vi "sub-GetLanguageInfo.vi"() -> (2 "selected":i32, 3 "languages":cluster{string, "appended path":path, string}[](array[cluster]))   [LabVIEW 2011]
uses:
  <vilib>/Utility/config.llb/Read Key (I32).vi
  <vilib>/Utility/config.llb/Read Key (String).vi
  <vilib>/Utility/config.llb/NI_LVConfig.lvlib
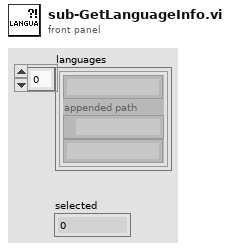
[diagram p1: front panel]
types:
  T1 = typedef "NI_LVConfig.lvlib/Config Data RefNum.ctl" = refnum<k1>
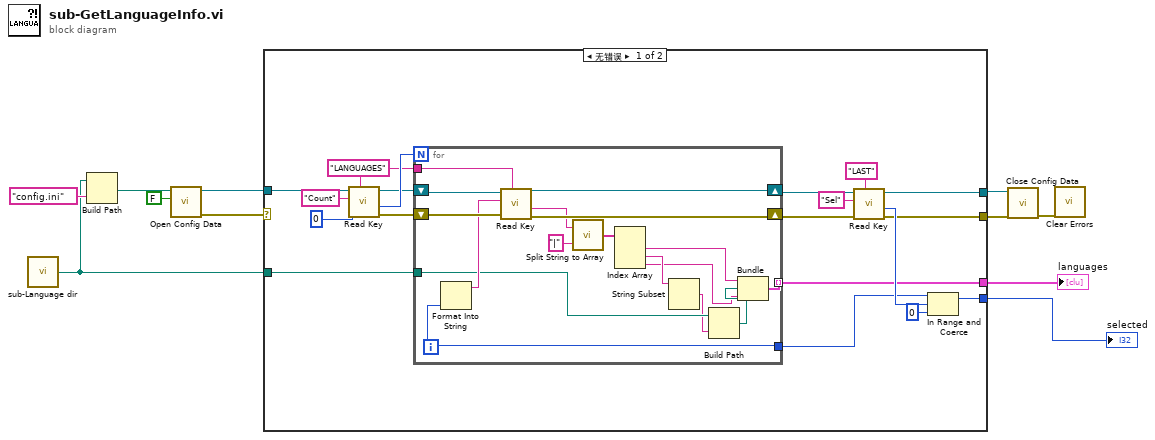
[diagram p0: block diagram]
diagram:
  n1 = call "sub-Language dir.vi"() -> ("folder"=w2:path)
  n2 = Build Path(base path=w2, name or relative path="config.ini" ("名称或相对路径")) -> (appended path=w10:path)
  n3 = call <vilib>:"Open Config Data.vi"("create file if necessary (T)"=FALSE, "configuration file path"=w10) -> ("error out"=w8:errorcluster, "refnum"=w7:T1)  [unwired: 7 in, 1 out]
  n4 = case shown="无错误" w8 {
    selector: w8 -> [_ w48]
    tunnel: w7 -> [w30 w49]
    tunnel: [w16 _] -> w3
    tunnel: [w15 _] -> w1
    tunnel: [w14 w49] -> w5
    tunnel: [w13 w48] -> w6
    tunnel: w2 -> [w12 _]
    frame No Error {
      w24 = "LANGUAGES" ("section")
      n5 = call-poly <vilib>:"Read Key.vi"("section"=w24, "default value"=0, "key"="Count", "refnum"=w30) -> ("error out"=w25:errorcluster, "value"=w27:i32, "refnum out"=w26:T1)  [unwired: 4 in, 1 out]
      n6 = for {
        N: w27 -> [_]
        shift-right: [w43] -> w23
        shift-left: w26 -> [w47]
        shift-right: [w42] -> w22
        shift-left: w25 -> [w46]
        tunnel: w24 -> [w45]
        tunnel: [w41] -> w15 mode=indexing
        tunnel: [w40] -> w18
        tunnel: w12 -> [w39]
        i -> [w40]
        n7 = Format Into String(w40) -> (resulting string=w44:string)  [unwired: 3 in, 1 out]
        n8 = call-poly <vilib>:"Read Key.vi"("section"=w45, "error in (no error)"=w46, "key"=w44, "refnum"=w47) -> ("error out"=w42:errorcluster, "value"=w36:string, "refnum out"=w43:T1)  [unwired: 4 in, 1 out]
        n9 = call "Split String to Array.vi"("搜索字符串/字符(-)"="|", "字符串"=w36) -> ("字符串数组"=w34:string[])
        n10 = Index Array(array=w34) -> (element #1=w33:string, element #2=w32:string, element #3=w31:string)  [unwired: 3 in]
        n11 = String Subset(string=w32) -> (substring=w38:string)  [unwired: 2 in]
        n12 = Build Path(base path=w39, name or relative path=w38) -> (appended path=w37:path)
        n13 = Bundle(w33, "appended path"=w37, w31) -> (w41:cluster{string, "appended path":path, string})  [unwired: 1 in]
      }
      n14 = call-poly <vilib>:"Read Key.vi"("section"="LAST", "error in (no error)"=w22, "key"="Sel", "refnum"=w23) -> ("error out"=w13:errorcluster, "value"=w19:i32, "refnum out"=w14:T1)  [unwired: 4 in, 1 out]
      n15 = In Range and Coerce(upper limit=w18, x=w19, lower limit=0 ("下限")) -> (coerced(x)=w16:i32)  [unwired: 1 out]
    }
    frame Error {
    }
  }
  "selected" <- w3
  "languages" <- w1
  n16 = call <vilib>:"Close Config Data.vi"("error in (no error)"=w6, "refnum"=w5) -> ("error out"=w4:errorcluster)  [unwired: 8 in, 1 out]
  n17 = call <vilib>:"Clear Errors.vi"("error in (no error)"=w4) -> ()  [unwired: 6 in, 1 out]
